vi "Update_Alarm_Panel.vi"(8 "error in (no error)":errorcluster, 10 "Data":variant, 11 "MHL_Data In":T1) -> (0 "error out":errorcluster, 3 "MHL_Data Out":T1)   [LabVIEW 2019, in "MHL.lvlib"]
uses:
  MHL.lvlib
  typedef/MHL_Data.ctl
  Alarm_Panel/Channel_Temperature_Threshold.ctl
  typedef/Alarm_Panel.ctl
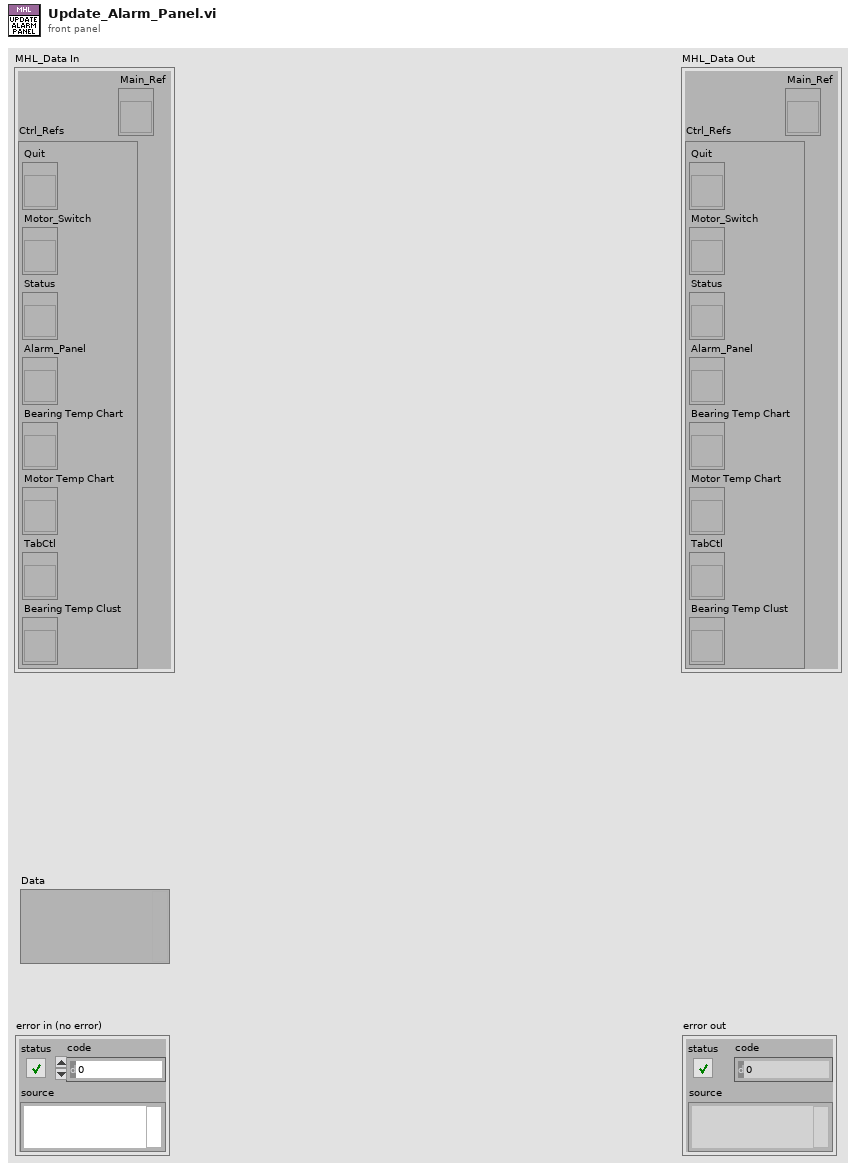
[diagram p1: front panel]
types:
  T1 = typedef "MHL.lvlib/MHL_Data.ctl" = cluster{"Ctrl_Refs":cluster{"Quit":refnum<vi>, "Motor_Switch":refnum<vi>, "Status":refnum<vi>, "Alarm_Panel":refnum<vi>, "Bearing Temp Chart":refnum<vi>, "Motor Temp Chart":refnum<vi>, "TabCtl":refnum<vi>, "Bearing Temp Clust":refnum<vi>}, "Main_Ref":refnum<vi>}
  T2 = typedef "Alarm_Panel.ctl" = cluster{"Channel (0 - 7)":cluster{"Channel Temperature Thresholds":T3, "Channel Temperature Thresholds 2":T3, "Channel Temperature Thresholds 3":T3, "Channel Temperature Thresholds 4":T3, "Channel Temperature Thresholds 5":T3, "Channel Temperature Thresholds 6":T3, "Channel Temperature Thresholds 7":T3, "Channel Temperature Thresholds 8":T3}, "Channel (8 - 15)":cluster{"Channel Temperature Thresholds":T3, "Channel Temperature Thresholds 2":T3, "Channel Temperature Thresholds 3":T3, "Channel Temperature Thresholds 4":T3, "Channel Temperature Thresholds 5":T3, "Channel Temperature Thresholds 6":T3, "Channel Temperature Thresholds 7":T3, "Channel Temperature Thresholds 8":T3}, "Channel (16 - 23)":cluster{"Channel Temperature Thresholds":T3, "Channel Temperature Thresholds 2":T3, "Channel Temperature Thresholds 3":T3, "Channel Temperature Thresholds 4":T3, "Channel Temperature Thresholds 5":T3, "Channel Temperature Thresholds 6":T3, "Channel Temperature Thresholds 7":T3, "Channel Temperature Thresholds 8":T3}, "Channel (24 - 31)":cluster{"Channel Temperature Thresholds":T3, "Channel Temperature Thresholds 2":T3, "Channel Temperature Thresholds 3":T3, "Channel Temperature Thresholds 4":T3, "Channel Temperature Thresholds 5":T3, "Channel Temperature Thresholds 6":T3, "Channel Temperature Thresholds 7":T3, "Channel Temperature Thresholds 8":T3}}
  T3 = typedef "Channel_Temperature_Threshold.ctl" = cluster{"Min":i32, "Max":i32, "Alarm":i32, "Status":u32}
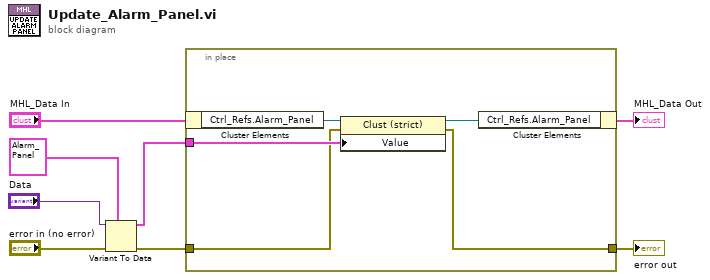
[diagram p0: block diagram]
diagram:
  n1 = Variant To Data(error in="error in (no error)", type=T2 {"Channel (0 - 7)"={"Channel Temperature Thresholds"={"Min"=0, "Max"=0, "Alarm"=0, "Status"=0}, "Channel Temperature Thresholds 2"={"Min"=0, "Max"=0, "Alarm"=0, "Status"=0}, "Channel Temperature Thresholds 3"={"Min"=0, "Max"=0, "Alarm"=0, "Status"=0}, "Channel Temperature Thresholds 4"={"Min"=0, "Max"=0, "Alarm"=0, "Status"=0}, "Channel Temperature Thresholds 5"={"Min"=0, "Max"=0, "Alarm"=0, "Status"=0}, "Channel Temperature Thresholds 6"={"Min"=0, "Max"=0, "Alarm"=0, "Status"=0}, "Channel Temperature Thresholds 7"={"Min"=0, "Max"=0, "Alarm"=0, "Status"=0}, "Channel Temperature Thresholds 8"={"Min"=0, "Max"=0, "Alarm"=0, "Status"=0}}, "Channel (8 - 15)"={"Channel Temperature Thresholds"={"Min"=0, "Max"=0, "Alarm"=0, "Status"=0}, "Channel Temperature Thresholds 2"={"Min"=0, "Max"=0, "Alarm"=0, "Status"=0}, "Channel Temperature Thresholds 3"={"Min"=0, "Max"=0, "Alarm"=0, "Status"=0}, "Channel Temperature Thresholds 4"={"Min"=0, "Max"=0, "Alarm"=0, "Status"=0}, "Channel Temperature Thresholds 5"={"Min"=0, "Max"=0, "Alarm"=0, "Status"=0}, "Channel Temperature Thresholds 6"={"Min"=0, "Max"=0, "Alarm"=0, "Status"=0}, "Channel Temperature Thresholds 7"={"Min"=0, "Max"=0, "Alarm"=0, "Status"=0}, "Channel Temperature Thresholds 8"={"Min"=0, "Max"=0, "Alarm"=0, "Status"=0}}, "Channel (16 - 23)"={"Channel Temperature Thresholds"={"Min"=0, "Max"=0, "Alarm"=0, "Status"=0}, "Channel Temperature Thresholds 2"={"Min"=0, "Max"=0, "Alarm"=0, "Status"=0}, "Channel Temperature Thresholds 3"={"Min"=0, "Max"=0, "Alarm"=0, "Status"=0}, "Channel Temperature Thresholds 4"={"Min"=0, "Max"=0, "Alarm"=0, "Status"=0}, "Channel Temperature Thresholds 5"={"Min"=0, "Max"=0, "Alarm"=0, "Status"=0}, "Channel Temperature Thresholds 6"={"Min"=0, "Max"=0, "Alarm"=0, "Status"=0}, "Channel Temperature Thresholds 7"={"Min"=0, "Max"=0, "Alarm"=0, "Status"=0}, "Channel Temperature Thresholds 8"={"Min"=0, "Max"=0, "Alarm"=0, "Status"=0}}, "Channel (24 - 31)"={"Channel Temperature Thresholds"={"Min"=0, "Max"=0, "Alarm"=0, "Status"=0}, "Channel Temperature Thresholds 2"={"Min"=0, "Max"=0, "Alarm"=0, "Status"=0}, "Channel Temperature Thresholds 3"={"Min"=0, "Max"=0, "Alarm"=0, "Status"=0}, "Channel Temperature Thresholds 4"={"Min"=0, "Max"=0, "Alarm"=0, "Status"=0}, "Channel Temperature Thresholds 5"={"Min"=0, "Max"=0, "Alarm"=0, "Status"=0}, "Channel Temperature Thresholds 6"={"Min"=0, "Max"=0, "Alarm"=0, "Status"=0}, "Channel Temperature Thresholds 7"={"Min"=0, "Max"=0, "Alarm"=0, "Status"=0}, "Channel Temperature Thresholds 8"={"Min"=0, "Max"=0, "Alarm"=0, "Status"=0}}} ("Alarm Panel"), Variant="Data") -> (data=w3:T2, error out=w1:errorcluster)
  n2 = in-place {
    in-place-border: w3 -> [w11]
    in-place-border: w1 -> [w10]
    in-place-border: [w9] -> w7
    n3 = in-place-cluster #1("MHL_Data In") -> ("Ctrl_Refs.Alarm_Panel"=w13:refnum<vi>)
    n4 = property class="Clust (strict)"(reference=w13, error in=w10, "Value"=w11) -> (reference out=w12:refnum<vi>, error out=w9:errorcluster)
    n5 = in-place-cluster #1("Ctrl_Refs.Alarm_Panel"=w12) -> (→"MHL_Data Out":T1)
  }
  "error out" <- w7
